vi "RS2323Portalicious.vi"() -> ()   [LabVIEW 2016]
uses:
  <vilib>/rvi/Emulation/niFpgaGetClockAttributes.vi
  <vilib>/rvi/Emulation/niFpgaSctlEmulationGetInTimedLoop.vi
  <vilib>/rvi/Emulation/niFpgaEmulationReportErrorSimple.vi
  <vilib>/rvi/eio/common/nirviEmuTemplateMethod_errors.vi
  <vilib>/rvi/Emulation/niFpgaCriticalErrorInLSC.vi
  <vilib>/eio/EIOMethodNode/EIOMethodNode.xnode
panel:
  out "Data":u8
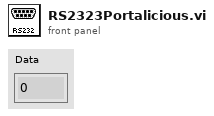
[diagram p1: front panel]
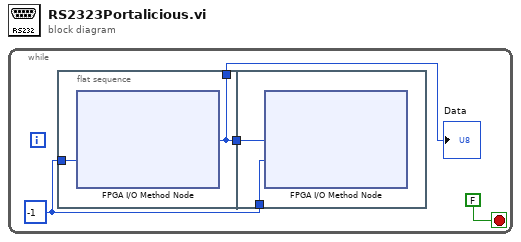
[diagram p0: block diagram]
diagram:
  n1 = while {
    stop <- FALSE stop-if-true
    w4 = i16 -1
    n2 = flat-sequence {
      tunnel: w4 -> [w6]
      tunnel: [w5] -> w2
      tunnel: [w5] -> w1
      tunnel: w4 -> [w8]
      tunnel: w2 -> [w7]
      frame #0 {
        n3 = xnode "FPGA I/O Method Node"("Timeout (ms)"=w6) -> ("Data"=w5:u8)  [unwired: 1 in, 2 out]
      }
      frame #1 {
        n4 = xnode "FPGA I/O Method Node"("Data"=w7, "Timeout (ms)"=w8) -> ()  [unwired: 1 in, 2 out]
      }
    }
    "Data" <- w1
  }
